vi "System_simulation.vi"() -> ()   [LabVIEW 2020]
uses:
  <vilib>/Simulation/Implementation/Shared/SIMSCR Execution Mode.ctl
  <vilib>/Simulation/Implementation/Shared/SIM Bundle Sim Info.vi
  <vilib>/Simulation/Implementation/Shared/SIM Unbundle Sim Info.vi
  <vilib>/Simulation/Implementation/Shared/NILVSim_FinalizeModel.vi
  <vilib>/Simulation/Implementation/Shared/NILVSim_GetModelError.vi
  <vilib>/Utility/error.llb/Clear Errors.vi
  <vilib>/Simulation/Implementation/Shared/SIMSH Read Queue.vi
  <vilib>/Simulation/Utility/Implementation/NILVSim Get Time and IsAcceptedStep.vi
  <vilib>/Simulation/Implementation/Shared/NILVSim_Manager.vi
  <vilib>/Simulation/Implementation/Shared/NILVSIM_BeginStep.vi
  <vilib>/Simulation/Implementation/Shared/NILVSim_Initialize.vi
  <vilib>/Simulation/Param Hierarchy/Typedefs/SIMPH Param Control Actions.ctl
  <vilib>/Simulation/Implementation/Shared/NILVSim_ParamChanged.vi
  <vilib>/Simulation/Scripting/Companion Diagram/SimConfigNode/SimParams.ctl
  <vilib>/Simulation/Scripting/Companion Diagram/SimConfigNode/_simSolvers.ctl
  <vilib>/Simulation/Implementation/XNodeFramework/SimXNode/SimX.xnode
  C:/Program Files/National Instruments/LabVIEW 2020/examples/Control and Simulation/Case Studies/Electrical Machines/DC Motor/SimEx DC Motor Model.vi
  <vilib>/Simulation/Implementation/Shared/NI_SIM_Implementation.lvlib
  <vilib>/Simulation/Scripting/Companion Diagram/SimConfigNode/SimDog.xnode
panel:
  out "Motor Torque":dbl(knob) scale=-10.0..10.0
  in  "Speed Voltage Factor":dbl=1.0 format="%#_13g"
  out "Motor Speed":dbl(knob) scale=-5.0..100.0
  in  "Motor Load":dbl(slide) scale=0.0..10.0
  out "Generator Speed":dbl(knob) scale=-5.0..100.0
  out "Generator Torque":dbl(knob) scale=-10.0..10.0
  in  "Initialize":bool
  in  "PWM":dbl(slide) scale=0.0..100.0
  in  "stop":bool
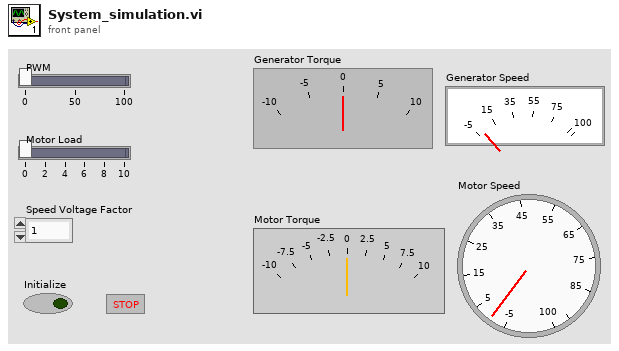
[diagram p1: front panel]
types:
  T1 = enum16{"Simulate to Completion", "Single Time-Step Simulation (Fixed Step Only)"}
  T2 = typedef "SIMSCR Execution Mode.ctl" = enum16{"Simulate to Completion", "Single Time-Step Simulation (Fixed Step Only)"}
  T3 = typedef "SIMPH Param Control Actions.ctl" = enum16{"get params", "set params"}
  T4 = cluster{"SIMSH Sim Time":dbl, "Integrator 6":cluster{"output":dbl}, "Gain 6":cluster{"output":dbl}, "Gain 5":cluster{"output":dbl}, "Gain 4":cluster{"output":dbl}, "Gain 3":cluster{"output":dbl}, "Gain 2":cluster{"output":dbl}, "Gain":cluster{"output":dbl}, "Integrator 4":cluster{"output":dbl}, "Summation 6":cluster{"Result":dbl}, "Summation 7":cluster{"Result":dbl}, "Integrator 5":cluster{"output":dbl}, "Unbundle By Name 2":cluster{"J":dbl, "Bm":dbl}, "Unbundle By Name":cluster{"Ra":dbl, "La":dbl}, "Reciprocal 2":cluster{"1/x":dbl}, "Reciprocal":cluster{"1/x":dbl}}
  T5 = typedef "SimParams.ctl" = cluster{"Initial Time (s)":dbl, "Final Time (s)":dbl, "Step Size (s)":dbl, "ODE Solver":T6, "Minimum Step Size (s)":dbl, "Maximum Step Size (s)":dbl, "Relative Tolerance":dbl, "Absolute Tolerance":dbl, "Software Timing":bool, "Initial Step Size (s)":dbl, "Automatic Fixed Step Size?":bool, "Automatic Discrete Step Size?":bool, "Discrete Step Size (s)":dbl, "Calculate using Time Step":bool, "Solver Wired?":bool, "Prev.Frm.Expected End":u64, "Prev.Frm.Actual End":u64, "Prev.Frm.Finished Late?":bool, "Prev.Iter.Expected End":u64, "Prev.Iter.Actual End":u64, "Prev.Iter.Finished Late?":bool, "Expected Iteration Start":u64, "Actual Iteration Start":u64, "Expected Frame Start":u64, "Actual Frame Start":u64, "Source Name":string, "Name":string, "Period":i64, "Deadline":i64, "Offset":i64, "Start":i64, "Priority":i32, "Timeout":i32, "Processor":i32, "Mode":enum32{"No Change", "Process missed periods, maintain original phase", "Discard missed periods, maintain original phase", "Process missed periods, ignore original phase", "Discard missed periods, ignore original phase"}, "Wakeup reason":enum32{"Normal", "Aborted", "Asynchronous wakeup", "Timing source error", "Timed loop error", "Timeout"}, "Error":errorcluster, "Source Type":string, "Secondary Source Type":string, "Global End Time":u64, "Global Start Time":u64, "Full Solver Reset":bool, "Execution Mode":T2, "Nan/Inf Check":bool, "Custom Solver Library":string, "Solver Is Variable":bool, "custom solver name":string, "Signal Collection Decimation":u32}
  T6 = typedef "_simSolvers.ctl" = enum16{"Runge-Kutta 1 (Euler)", "Runge-Kutta 2", "Runge-Kutta 3", "Runge-Kutta 4", "Runge-Kutta 23 (variable)", "Runge-Kutta 45 (variable)", "BDF (variable)", "Adams-Moulton (variable)", "Rosenbrock (variable)", "Discrete States Only", "SDIRK 4 (variable)", "Radau 5 (variable)", "Radau 9 (variable)", "Radau 13 (variable)", "Radau [Variable Order] (variable)", "Gear's Method (variable)", "Linearizer", "State Query", "Trim Eval", "Custom Solver"}
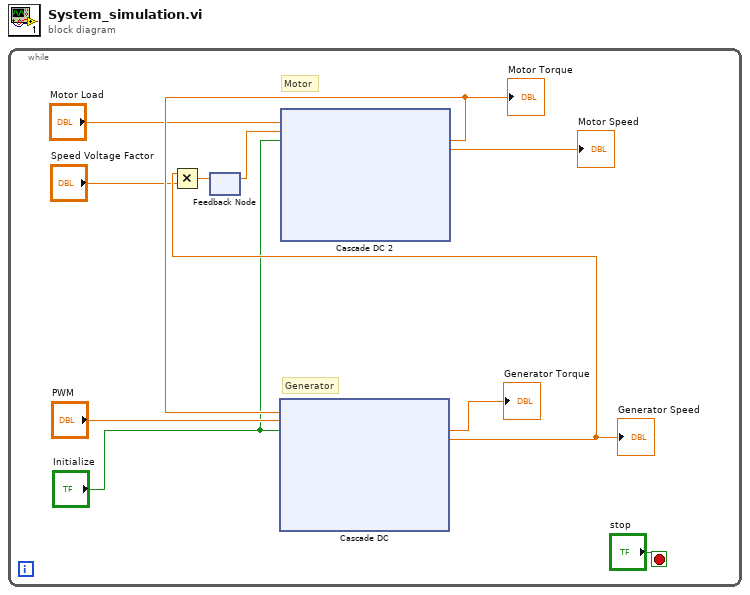
[diagram p0: block diagram]
diagram:
  n1 = while {
    stop <- "stop" stop-if-true
    # "Generator"
    # "Motor"
    n2 = feedback #1() -> (w3:dbl)  [unwired: 1 in]
    n3 = xnode ("Cascade DC 2")("TL"="Motor Load", "voltage"=w3, "Initialize"="Initialize") -> ("Te"=w8:dbl, "Speed"=→"Motor Speed":dbl)  [unwired: 1 in, 6 out]
    "Motor Torque" <- w8
    n4 = xnode ("Cascade DC")("TL"=w8, "voltage"="PWM", "Initialize"="Initialize") -> ("Te"=→"Generator Torque":dbl, "Speed"=w6:dbl)  [unwired: 1 in, 6 out]
    "Generator Speed" <- w6
    n5 = Multiply(x=w6, y="Speed Voltage Factor") -> (x*y=w4:dbl)
    n6 = feedback-in #1(w4) -> ()
  }
